vi "Open Protocol.vi"(8 "error in (no error)":errorcluster, 11 "Time Protocol in":refnum<class "Time Protocol.lvclass">) -> (0 "error out":errorcluster, 3 "Time Protocol out":refnum<class "Time Protocol.lvclass">)   [LabVIEW 2012, in "Time Protocol Actor.lvlib" / "Time Protocol.lvclass"]
uses:
  Time Protocol.lvclass
  Time Protocol.lvclass/Time Protocol.ctl
  Read History.vi
  Read Code.vi
  Read Path.vi
  Read Open.vi
  <vilib>/Utility/file.llb/Read From Spreadsheet File (string).vi
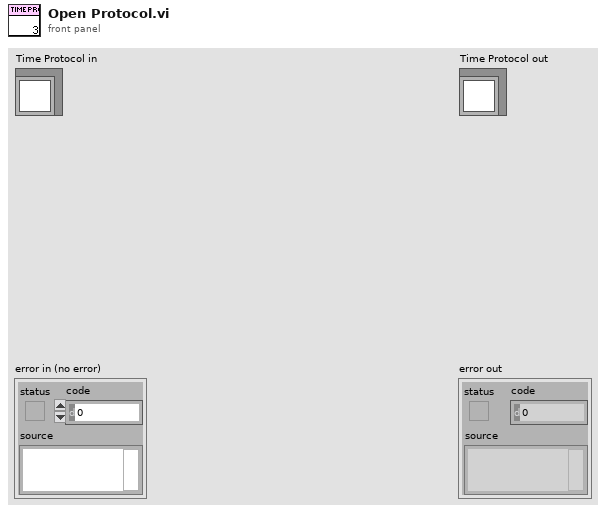
[diagram p1: front panel]
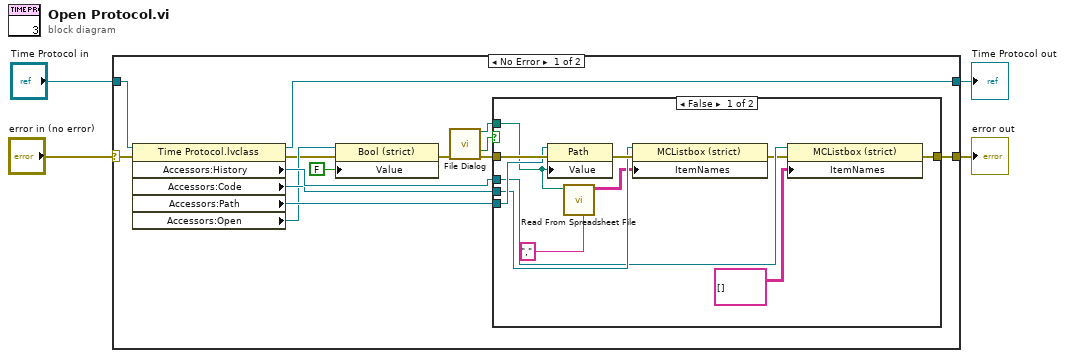
[diagram p0: block diagram]
diagram:
  n1 = case shown="No Error" "error in (no error)" {
    selector: "error in (no error)" -> [w6 w32]
    tunnel: [w5 w32] -> w3
    tunnel: [w12 w31] -> w1
    tunnel: "Time Protocol in" -> [w13 w31]
    frame No Error {
      n2 = property class="Time Protocol.lvclass"(reference=w13, error in=w6) -> (reference out=w12:refnum<class "Time Protocol.lvclass">, error out=w7:errorcluster, "Accessors:History"=w11:refnum<vi>, "Accessors:Code"=w10:refnum<vi>, "Accessors:Path"=w9:refnum<vi>, "Accessors:Open"=w8:refnum<vi>)
      n3 = property class="Bool (strict)"(reference=w8, error in=w7, "Value"=FALSE) -> (error out=w16:errorcluster)  [unwired: 1 out]
      n4 = call "File Dialog"("error in"=w16) -> ("selected path"=w17:path, "cancelled"=w14:bool, "error out"=w18:errorcluster)  [unwired: 11 in, 1 out]
      n5 = case shown="False" w14 {
        tunnel: w10 -> [w24 _]
        tunnel: w18 -> [w28 w30]
        tunnel: w9 -> [w27 _]
        tunnel: w17 -> [w26 _]
        tunnel: [w19 w30] -> w5
        tunnel: w11 -> [w22 _]
        frame False {
          n6 = property class="Path"(reference=w27, error in=w28, "Value"=w26) -> (error out=w25:errorcluster)  [unwired: 1 out]
          n7 = call-poly <vilib>:"Read From Spreadsheet File.vi"("delimiter (\\t)"="," ("delimiter (\\t)"), "file path (dialog if empty)"=w26) -> ("all rows"=w23:string[][])  [unwired: 5 in, 4 out]
          n8 = property class="MCListbox (strict)"(reference=w24, error in=w25, "ItemNames"=w23) -> (error out=w21:errorcluster)  [unwired: 1 out]
          n9 = property class="MCListbox (strict)"(reference=w22, error in=w21, "ItemNames"=string[][] [] ("Item Names")) -> (error out=w19:errorcluster)  [unwired: 1 out]
        }
        frame True {
        }
      }
    }
    frame Error {
    }
  }
  "error out" <- w3
  "Time Protocol out" <- w1
